vi "1.0.2_UUT_Reflashing.vi"(8 "error in (no error)":errorcluster, 10 "Data in":T1, 11 "Message Queue out":T2) -> (0 "error out":errorcluster, 1 "Flow":string, 2 "Data out":T1, 3 "Message Queue Out":T2)   [LabVIEW 2017]
uses:
  Depends/AMC/subVIs/TypeDefs/amc_Message Queue.ctl
  Depends/AMC/subVIs/TypeDefs/amc_Message.ctl
  Depends/Tools/Keyed Array/Tools_KeyedArray KeyedArray.ctl
  Ctrls/CSV_Data.ctl
  DIPC 692 Daemon API/typdef/destination.ctl
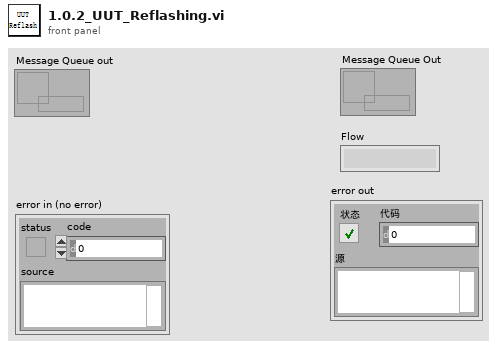
[diagram p1: front panel]
types:
  T1 = typedef "CSV_Data.ctl" = cluster{"Initialisation":cluster{"LMT - Connect UUT (con COM)":string, "LMT - Software Version (rrel)":string, "LMT - Write SKU file (wskuc)":string, "LMT - SKU file name":string, "Connect UUT DDM":string, "Read DDM EOL Timestamp - Mode":string, "Read DDM EOL Timestamp - Timestamp":string, "Read DDM EOL Timestamp - Rig ID":string, "Read DDM EOL Timestamp - Passmark ID":string, "Read DDM EOL Timestamp - Passmark Rev":string, "Software Version before flashing":string, "Read Hardware Serial":string, "UUT DDM SN":string, "Compare DDM SN with MES SN":string, "Backup PCBA Calibration EEPROM Response - CAL":string, "Flash Firmware Version":string, "Check SW Version":string, "Read DDM SW Version after flashing":string, "Set SKU Config":string, "Ready Status":string, "Set Device Mode to EOL":string, "DDM Parameter - Voltage":string, "DDM Parameter - Current":string, "DDM Parameter - Power":string, "DDM Parameter - Speed":string, "DDM Parameter - Pressure":string, "Tester Parameter - Voltage":string, "Tester Parameter - Current":string, "Tester Parameter - Power":string, "Tester Parameter - Ambient Pressure":string, "Tester Parameter - Ambient Temperature":string, "Calculated Parameter - DDM Pressure Corrected":string, "Calculated Parameter - DDM Real Power":string, "Calculated Parameter - Delta V":string}, "BEMF_Calibration":cluster{"Calibration Result - eol_cold_bemf_temp":string, "DDM Ambient Temp":string, "Restriction Plate Diameter":string, "Calibration Result - eol_bemf_mp_cold_coef_a":string, "Calibration Result - eol_bemf_mp_cold_coef_b":string, "Calibration Result - eol_bemf_mp_cold_coef_c":string, "Calibration Result - eol_bemf_lsi_cold_ref_coeffs":string, "Get - Calibration Result - eol_bemf_lsi_speed":string, "Get - Calibration Result - eol_bemf_lsi_integral_0":string, "Calibration Result - eol_bemf_lsi_integral_1":string, "Get - Calibration Result - eol_bemf_lsi_integral_2":string, "Get - Calibration Result - eol_cold_bemf":string, "Get - Calibration Result - eol_cold_bemf_fisf":string, "Finalise Calibration":string, "Compare -Calibration Result - eol_cold_bemf":string, "Compare -Calibration Result - eol_cold_bemf_fisf":string}, "ECO":cluster{"Reset Power Tune":string, "Reset BEMF FISF Calibration":string, "Restriction Plate Diameter":string, "ECO - Stabilisation Time":string, "ECO - DDM Parameter - Voltage":string, "ECO - DDM Parameter - Current":string, "ECO - DDM Parameter - Power":string, "ECO - DDM Parameter - Measured Power":string, "ECO - DDM Parameter - Speed":string, "ECO - DDM Parameter - Pressure":string, "ECO - Tester Parameter - Voltage":string, "ECO - Tester Parameter - Current":string, "ECO - Tester Parameter - Power":string, "ECO - Tester Parameter - Ambient Pressure":string, "ECO - Tester Parameter - Ambient Temperature":string, "ECO - Tester Parameter - Ambient Humidity":string, "ECO - Calculated Parameter - DDM Pressure Corrected":string, "ECO - Calculated Parameter - DDM Real Power":string, "ECO - Calculated Parameter - Delta V":string, "ECO - Calculated Parameter - Flowrate":string, "ECO - Calculated Parameter - Airwatt":string, "ECO - Formula":string, "PT ECO - Power Tune Mode Status":string}, "BOOST":cluster{"Restriction Plate Diameter":string, "BOOST - Stabilisation Time":string, "BOOST - DDM Parameter - Voltage":string, "BOOST - DDM Parameter - Current":string, "BOOST - DDM Parameter - Power":string, "BOOST - DDM Parameter - Measured Power":string, "BOOST - DDM Parameter - Speed":string, "BOOST - DDM Parameter - Pressure":string, "BOOST - Tester Parameter - Voltage":string, "BOOST - Tester Parameter - Current":string, "BOOST - Tester Parameter - Power":string, "BOOST - Tester Parameter - Ambient Pressure":string, "BOOST - Tester Parameter - Ambient Temperature":string, "BOOST - Tester Parameter - Ambient Humidity":string, "BOOST - Calculated Parameter - DDM Pressure Corrected":string, "BOOST - Calculated Parameter - DDM Real Power":string, "BOOST - Calculated Parameter - Delta V":string, "BOOST - Calculated Parameter - Flowrate":string, "BOOST - Calculated Parameter - Airwatt":string, "BOOST - Get AM Presence":string, "Air Muscle Turn Off Status":string, "BOOST - Air Muscle Calculated Parameter - Airwatt B":string, "BOOST - Air Muscle Calculate Airwatt Delta":string, "PT BOOST - Power Tune Mode Status":string, "Finalise Calibration":string, "ECO - Get AW Calibration value":string, "BOOST - Get AW Calibration value":string}, "MAX":cluster{"Restriction Plate Diameter":string, "MAX - Stabilisation Time":string, "Get Average Delta Tmag (LSIdelta_FISFdelta_LSItmag_FISFtmag_IIRtmag)":string, "Get Average Delta Tmag FISF":string, "MAX - DDM Parameter - Voltage":string, "MAX - DDM Parameter - Current":string, "MAX - DDM Parameter - Power":string, "MAX - DDM Parameter - Measured Power":string, "MAX - DDM Parameter - Speed":string, "MAX - DDM Parameter - Pressure":string, "MAX - Tester Parameter - Voltage":string, "MAX - Tester Parameter - Current":string, "MAX - Tester Parameter - Power":string, "MAX - Tester Parameter - Ambient Pressure":string, "MAX - Tester Parameter - Ambient Temperature":string, "MAX - Tester Parameter - Ambient Humidity":string, "MAX - Calculated Parameter - DDM Pressure Corrected":string, "MAX - Calculated Parameter - DDM Real Power":string, "MAX - Calculated Parameter - Delta V":string, "MAX - Calculated Parameter - Flowrate":string, "MAX - Calculated Parameter - Airwatt":string, "MAX_FISF_Check_Average_Delta_Tmag":string, "MAX - FISF - BEMF Finetune Result":string, "MAX tune - Delta P1":string, "MAX tune - Calculated Parameter - Airwatt":string, "Calculate Delta Airwatts - MAX finetune - Delta P2":string, "MAX finetune - DDM Parameter - Voltage":string, "MAX finetune - DDM Parameter - Current":string, "MAX finetune - DDM Parameter - Power":string, "MAX finetune - DDM Parameter - Measured Power":string, "MAX finetune - DDM Parameter - Speed":string, "MAX finetune - DDM Parameter - Pressure":string, "MAX finetune - Tester Parameter - Voltage":string, "MAX finetune - Tester Parameter - Current":string, "MAX finetune - Tester Parameter - Power":string, "MAX finetune - Tester Parameter - Ambient Pressure":string, "MAX finetune - Tester Parameter - Ambient Temperature":string, "MAX finetune - Tester Parameter - Ambient Humidity":string, "MAX finetune - Calculated Parameter - DDM Pressure Corrected":string, "MAX finetune - Calculated Parameter - DDM Real Power":string, "MAX finetune - Calculated Parameter - Delta V":string, "MAX finetune - Calculated Parameter - Flowrate":string, "MAX finetune - Calculated Parameter - Airwatt":string, "Check Derate Result":string, "Delta Tmag FISF":string, "Get Hot BEMF Result":string, "Calculate delta Pressure":string, "Finalise Calibration":string, "Calculate & Check Delta BEMF":string, "Delta P Airwatts Value":string}, "LL":cluster{"DDM Ambient Temp":string, "Restriction Plate Diameter":string, "LL - DDM Parameter - Voltage":string, "LL - DDM Parameter - Current":string, "LL - DDM Parameter - Power":string, "LL - DDM Parameter - Measured Power":string, "LL - DDM Parameter - Speed":string, "LL - DDM Parameter - Pressure":string, "LL - Tester Parameter - Voltage":string, "LL - Tester Parameter - Current":string, "LL - Tester Parameter - Power":string, "LL - DDM Real Power":string, "LL - Calibrate Task Detect LL":string}, "HL":cluster{"HL - DDM Parameter - Voltage":string, "HL - DDM Parameter - Current":string, "HL - DDM Parameter - Power":string, "HL - DDM Parameter - Measured Power":string, "HL - DDM Parameter - Speed":string, "HL - DDM Parameter - Pressure":string, "HL - Tester Parameter - Voltage":string, "HL - Tester Parameter - Current":string, "HL - Tester Parameter - Power":string, "HL - DDM Real Power":string, "HL - Calibrate Task Detect HL":string}, "LH":cluster{"Restriction Plate Diameter":string, "LH - DDM Parameter - Voltage":string, "LH - DDM Parameter - Current":string, "LH - DDM Parameter - Power":string, "LH - DDM Parameter - Measured Power":string, "LH - DDM Parameter - Speed":string, "LH - DDM Parameter - Pressure":string, "LH - Tester Parameter - Voltage":string, "LH - Tester Parameter - Current":string, "LH - Tester Parameter - Power":string, "LH - DDM Real Power":string, "LH - Calibrate Task Detect LH":string}, "HH":cluster{"HH - DDM Parameter - Voltage":string, "HH - DDM Parameter - Current":string, "HH - DDM Parameter - Power":string, "HH - DDM Parameter - Measured Power":string, "HH - DDM Parameter - Speed":string, "HH - DDM Parameter - Pressure":string, "HH - Tester Parameter - Voltage":string, "HH - Tester Parameter - Current":string, "HH - Tester Parameter - Power":string, "HH - DDM Real Power":string, "HH - Calibrate Task Detect HH":string}, "Inlet Blockage Calibration":cluster{"Inlet Blockage Calibration - DDM Parameter - Voltage":string, "Inlet Blockage Calibration - DDM Parameter - Current":string, "Inlet Blockage Calibration - DDM Parameter - Power":string, "Inlet Blockage Calibration - DDM Parameter - Measured Power":string, "Inlet Blockage Calibration - DDM Parameter - Speed":string, "Inlet Blockage Calibration - DDM Parameter - Pressure":string, "Inlet Blockage Calibration - Tester Parameter - Voltage":string, "Inlet Blockage Calibration - Tester Parameter - Current":string, "Inlet Blockage Calibration - Tester Parameter - Power":string, "Inlet Blockage Calibration - DDM Real Power":string, "Calibration Inlet Blockage_E":string, "Finalise Calibration":string, "Get Task Detect LL":string, "Get Task Detect HL":string, "Get Task Detect LH":string, "Get Task Detect HH":string, "Calibration Inlet Blockage":string, "Calibration eol cold bemf temp":string}, "GOOD":cluster{"GOOD UNIT - Clear EEPROM Error Log":string, "GOOD UNIT - Write Product Timestamp - Mode":string, "GOOD UNIT - Write Product Timestamp - Timestamp":string, "GOOD UNIT - Write Product Timestamp - Rig ID":string, "GOOD UNIT - Write Product Timestamp - Passmark ID":string, "GOOD UNIT - Write Product Timestamp - Passmark Rev":string, "GOOD UNIT - Set Device Mode to PROD":string, "GOOD UNIT - Backup PCBA Calibration EEPROM Response":string, "GOOD UNIT - Check Security Bit":string, "GOOD UNIT - Set Calibration Lock":string, "GOOD UNIT - Get_Calibration_Lock":string, "GOOD UNIT - Disconnect UUT":string}, "NG":cluster{"NG UNIT - Read NVM Error":string, "NG UNIT - Set Device Mode to FCT":string, "NG UNIT - Backup PCBA Calibration EEPROM Response - CAL":string, "NG UNIT - Backup PCBA Calibration EEPROM Response - ERROR":string, "NG UNIT - Backup PCBA Calibration EEPROM Response - USAGE":string, "NG UNIT - Disconnect UUT":string}, "SN":string, "Table":string[][], "Count":cluster{"Total":i32, "OK":i32, "NG":i32, "Yield":dbl}, "Start Time":timestamp, "daemon reference":refnum<k5>, "CT":dbl, "Config":string[][], "OK/NG":bool, "Station ID":string, "MES DDM SN":string, "MES PCBA SN":string, "Retest":string, "Lux":string, "Initialisation_Status":cluster{"LMT - Connect UUT (con COM)":string, "LMT - Software Version (rrel)":string, "LMT - Write SKU file (wskuc)":string, "LMT - SKU file name":string, "Connect UUT DDM":string, "Read DDM EOL Timestamp - Mode":string, "Read DDM EOL Timestamp - Timestamp":string, "Read DDM EOL Timestamp - Rig ID":string, "Read DDM EOL Timestamp - Passmark ID":string, "Read DDM EOL Timestamp - Passmark Rev":string, "Software Version before flashing":string, "Read Hardware Serial":string, "UUT DDM SN":string, "Compare DDM SN with MES SN":string, "Backup PCBA Calibration EEPROM Response - CAL":string, "Flash Firmware Version":string, "Check SW Version":string, "Read DDM SW Version after flashing":string, "Set SKU Config":string, "Ready Status":string, "Set Device Mode to EOL":string, "DDM Parameter - Voltage":string, "DDM Parameter - Current":string, "DDM Parameter - Power":string, "DDM Parameter - Speed":string, "DDM Parameter - Pressure":string, "Tester Parameter - Voltage":string, "Tester Parameter - Current":string, "Tester Parameter - Power":string, "Tester Parameter - Ambient Pressure":string, "Tester Parameter - Ambient Temperature":string, "Calculated Parameter - DDM Pressure Corrected":string, "Calculated Parameter - DDM Real Power":string, "Calculated Parameter - Delta V":string}, "BEMF_Calibration_Status":cluster{"Calibration Result - eol_cold_bemf_temp":string, "DDM Ambient Temp":string, "Restriction Plate Diameter":string, "Calibration Result - eol_bemf_mp_cold_coef_a":string, "Calibration Result - eol_bemf_mp_cold_coef_b":string, "Calibration Result - eol_bemf_mp_cold_coef_c":string, "Calibration Result - eol_bemf_lsi_cold_ref_coeffs":string, "Get - Calibration Result - eol_bemf_lsi_speed":string, "Get - Calibration Result - eol_bemf_lsi_integral_0":string, "Calibration Result - eol_bemf_lsi_integral_1":string, "Get - Calibration Result - eol_bemf_lsi_integral_2":string, "Get - Calibration Result - eol_cold_bemf":string, "Get - Calibration Result - eol_cold_bemf_fisf":string, "Finalise Calibration":string, "Compare -Calibration Result - eol_cold_bemf":string, "Compare -Calibration Result - eol_cold_bemf_fisf":string}, "ECO_Status":cluster{"Reset Power Tune":string, "Reset BEMF FISF Calibration":string, "Restriction Plate Diameter":string, "ECO - Stabilisation Time":string, "ECO - DDM Parameter - Voltage":string, "ECO - DDM Parameter - Current":string, "ECO - DDM Parameter - Power":string, "ECO - DDM Parameter - Measured Power":string, "ECO - DDM Parameter - Speed":string, "ECO - DDM Parameter - Pressure":string, "ECO - Tester Parameter - Voltage":string, "ECO - Tester Parameter - Current":string, "ECO - Tester Parameter - Power":string, "ECO - Tester Parameter - Ambient Pressure":string, "ECO - Tester Parameter - Ambient Temperature":string, "ECO - Tester Parameter - Ambient Humidity":string, "ECO - Calculated Parameter - DDM Pressure Corrected":string, "ECO - Calculated Parameter - DDM Real Power":string, "ECO - Calculated Parameter - Delta V":string, "ECO - Calculated Parameter - Flowrate":string, "ECO - Calculated Parameter - Airwatt":string, "ECO - Formula":string, "PT ECO - Power Tune Mode Status":string}, "BOOST_Status":cluster{"Restriction Plate Diameter":string, "BOOST - Stabilisation Time":string, "BOOST - DDM Parameter - Voltage":string, "BOOST - DDM Parameter - Current":string, "BOOST - DDM Parameter - Power":string, "BOOST - DDM Parameter - Measured Power":string, "BOOST - DDM Parameter - Speed":string, "BOOST - DDM Parameter - Pressure":string, "BOOST - Tester Parameter - Voltage":string, "BOOST - Tester Parameter - Current":string, "BOOST - Tester Parameter - Power":string, "BOOST - Tester Parameter - Ambient Pressure":string, "BOOST - Tester Parameter - Ambient Temperature":string, "BOOST - Tester Parameter - Ambient Humidity":string, "BOOST - Calculated Parameter - DDM Pressure Corrected":string, "BOOST - Calculated Parameter - DDM Real Power":string, "BOOST - Calculated Parameter - Delta V":string, "BOOST - Calculated Parameter - Flowrate":string, "BOOST - Calculated Parameter - Airwatt":string, "BOOST - Get AM Presence":string, "Air Muscle Turn Off Status":string, "BOOST - Air Muscle Calculated Parameter - Airwatt B":string, "BOOST - Air Muscle Calculate Airwatt Delta":string, "PT BOOST - Power Tune Mode Status":string, "Finalise Calibration":string, "ECO - Get AW Calibration value":string, "BOOST - Get AW Calibration value":string}, "MAX_Status":cluster{"Restriction Plate Diameter":string, "MAX - Stabilisation Time":string, "Get Average Delta Tmag (LSIdelta_FISFdelta_LSItmag_FISFtmag_IIRtmag)":string, "Get Average Delta Tmag FISF":string, "MAX - DDM Parameter - Voltage":string, "MAX - DDM Parameter - Current":string, "MAX - DDM Parameter - Power":string, "MAX - DDM Parameter - Measured Power":string, "MAX - DDM Parameter - Speed":string, "MAX - DDM Parameter - Pressure":string, "MAX - Tester Parameter - Voltage":string, "MAX - Tester Parameter - Current":string, "MAX - Tester Parameter - Power":string, "MAX - Tester Parameter - Ambient Pressure":string, "MAX - Tester Parameter - Ambient Temperature":string, "MAX - Tester Parameter - Ambient Humidity":string, "MAX - Calculated Parameter - DDM Pressure Corrected":string, "MAX - Calculated Parameter - DDM Real Power":string, "MAX - Calculated Parameter - Delta V":string, "MAX - Calculated Parameter - Flowrate":string, "MAX - Calculated Parameter - Airwatt":string, "MAX_FISF_Check_Average_Delta_Tmag":string, "MAX - FISF - BEMF Finetune Result":string, "MAX tune - Delta P1":string, "MAX tune - Calculated Parameter - Airwatt":string, "Calculate Delta Airwatts - MAX finetune - Delta P2":string, "MAX finetune - DDM Parameter - Voltage":string, "MAX finetune - DDM Parameter - Current":string, "MAX finetune - DDM Parameter - Power":string, "MAX finetune - DDM Parameter - Measured Power":string, "MAX finetune - DDM Parameter - Speed":string, "MAX finetune - DDM Parameter - Pressure":string, "MAX finetune - Tester Parameter - Voltage":string, "MAX finetune - Tester Parameter - Current":string, "MAX finetune - Tester Parameter - Power":string, "MAX finetune - Tester Parameter - Ambient Pressure":string, "MAX finetune - Tester Parameter - Ambient Temperature":string, "MAX finetune - Tester Parameter - Ambient Humidity":string, "MAX finetune - Calculated Parameter - DDM Pressure Corrected":string, "MAX finetune - Calculated Parameter - DDM Real Power":string, "MAX finetune - Calculated Parameter - Delta V":string, "MAX finetune - Calculated Parameter - Flowrate":string, "MAX finetune - Calculated Parameter - Airwatt":string, "Check Derate Result":string, "Delta Tmag FISF":string, "Get Hot BEMF Result":string, "Calculate delta Pressure":string, "Finalise Calibration":string, "Calculate & Check Delta BEMF":string, "Delta P Airwatts Value":string}, "LL_Status":cluster{"DDM Ambient Temp":string, "Restriction Plate Diameter":string, "LL - DDM Parameter - Voltage":string, "LL - DDM Parameter - Current":string, "LL - DDM Parameter - Power":string, "LL - DDM Parameter - Measured Power":string, "LL - DDM Parameter - Speed":string, "LL - DDM Parameter - Pressure":string, "LL - Tester Parameter - Voltage":string, "LL - Tester Parameter - Current":string, "LL - Tester Parameter - Power":string, "LL - DDM Real Power":string, "LL - Calibrate Task Detect LL":string}, "HL_Status":cluster{"HL - DDM Parameter - Voltage":string, "HL - DDM Parameter - Current":string, "HL - DDM Parameter - Power":string, "HL - DDM Parameter - Measured Power":string, "HL - DDM Parameter - Speed":string, "HL - DDM Parameter - Pressure":string, "HL - Tester Parameter - Voltage":string, "HL - Tester Parameter - Current":string, "HL - Tester Parameter - Power":string, "HL - DDM Real Power":string, "HL - Calibrate Task Detect HL":string}, "LH_Status":cluster{"Restriction Plate Diameter":string, "LH - DDM Parameter - Voltage":string, "LH - DDM Parameter - Current":string, "LH - DDM Parameter - Power":string, "LH - DDM Parameter - Measured Power":string, "LH - DDM Parameter - Speed":string, "LH - DDM Parameter - Pressure":string, "LH - Tester Parameter - Voltage":string, "LH - Tester Parameter - Current":string, "LH - Tester Parameter - Power":string, "LH - DDM Real Power":string, "LH - Calibrate Task Detect LH":string}, "HH_Status":cluster{"HH - DDM Parameter - Voltage":string, "HH - DDM Parameter - Current":string, "HH - DDM Parameter - Power":string, "HH - DDM Parameter - Measured Power":string, "HH - DDM Parameter - Speed":string, "HH - DDM Parameter - Pressure":string, "HH - Tester Parameter - Voltage":string, "HH - Tester Parameter - Current":string, "HH - Tester Parameter - Power":string, "HH - DDM Real Power":string, "HH - Calibrate Task Detect HH":string}, "Inlet Blockage Calibration_Status":cluster{"Inlet Blockage Calibration - DDM Parameter - Voltage":string, "Inlet Blockage Calibration - DDM Parameter - Current":string, "Inlet Blockage Calibration - DDM Parameter - Power":string, "Inlet Blockage Calibration - DDM Parameter - Measured Power":string, "Inlet Blockage Calibration - DDM Parameter - Speed":string, "Inlet Blockage Calibration - DDM Parameter - Pressure":string, "Inlet Blockage Calibration - Tester Parameter - Voltage":string, "Inlet Blockage Calibration - Tester Parameter - Current":string, "Inlet Blockage Calibration - Tester Parameter - Power":string, "Inlet Blockage Calibration - DDM Real Power":string, "Calibration Inlet Blockage_E":string, "Finalise Calibration":string, "Get Task Detect LL":string, "Get Task Detect HL":string, "Get Task Detect LH":string, "Get Task Detect HH":string, "Calibration Inlet Blockage":string, "Calibration eol cold bemf temp":string}, "GOOD_Status":cluster{"GOOD UNIT - Clear EEPROM Error Log":string, "GOOD UNIT - Write Product Timestamp - Mode":string, "GOOD UNIT - Write Product Timestamp - Timestamp":string, "GOOD UNIT - Write Product Timestamp - Rig ID":string, "GOOD UNIT - Write Product Timestamp - Passmark ID":string, "GOOD UNIT - Write Product Timestamp - Passmark Rev":string, "GOOD UNIT - Set Device Mode to PROD":string, "GOOD UNIT - Backup PCBA Calibration EEPROM Response":string, "GOOD UNIT - Check Security Bit":string, "GOOD UNIT - Set Calibration Lock":string, "GOOD UNIT - Get_Calibration_Lock":string, "GOOD UNIT - Disconnect UUT":string}, "NG_Status":cluster{"NG UNIT - Read NVM Error":string, "NG UNIT - Set Device Mode to FCT":string, "NG UNIT - Backup PCBA Calibration EEPROM Response - CAL":string, "NG UNIT - Backup PCBA Calibration EEPROM Response - ERROR":string, "NG UNIT - Backup PCBA Calibration EEPROM Response - USAGE":string, "NG UNIT - Disconnect UUT":string}, "SKU":string, "Plate_Diameter":string, "Alarm":string}
  T2 = typedef "amc_Message Queue.ctl" = refnum<queue>
  T3 = typedef "HD Config.ctl" = cluster{" PC":cluster{"PC Address":u8[], "PC Port":i32}, "FCO":cluster{"COM":refnum<visa-resource-name>, "Baudrate":u32}, "DC Power ":cluster{"COM":refnum<visa-resource-name>, "Baudrate":u32}, "PW3336":cluster{"COM":refnum<visa-resource-name>, "Baudrate":u32}, "Lefoo":cluster{"COM":refnum<visa-resource-name>, "Baudrate":u32}, "Tempt&Hum":cluster{"COM":refnum<visa-resource-name>, "Baudrate":u32}, "DIPC":cluster{"COM":refnum<visa-resource-name>}, "Daemon":cluster{"IP Address":string, "Port":u16, "Retry":u16}, "NFC":cluster{"COM":refnum<visa-resource-name>, "Baudrate":u32}, "Fail_resume_mode":bool, "GRR":bool}
  T4 = typedef "destination.ctl" = string
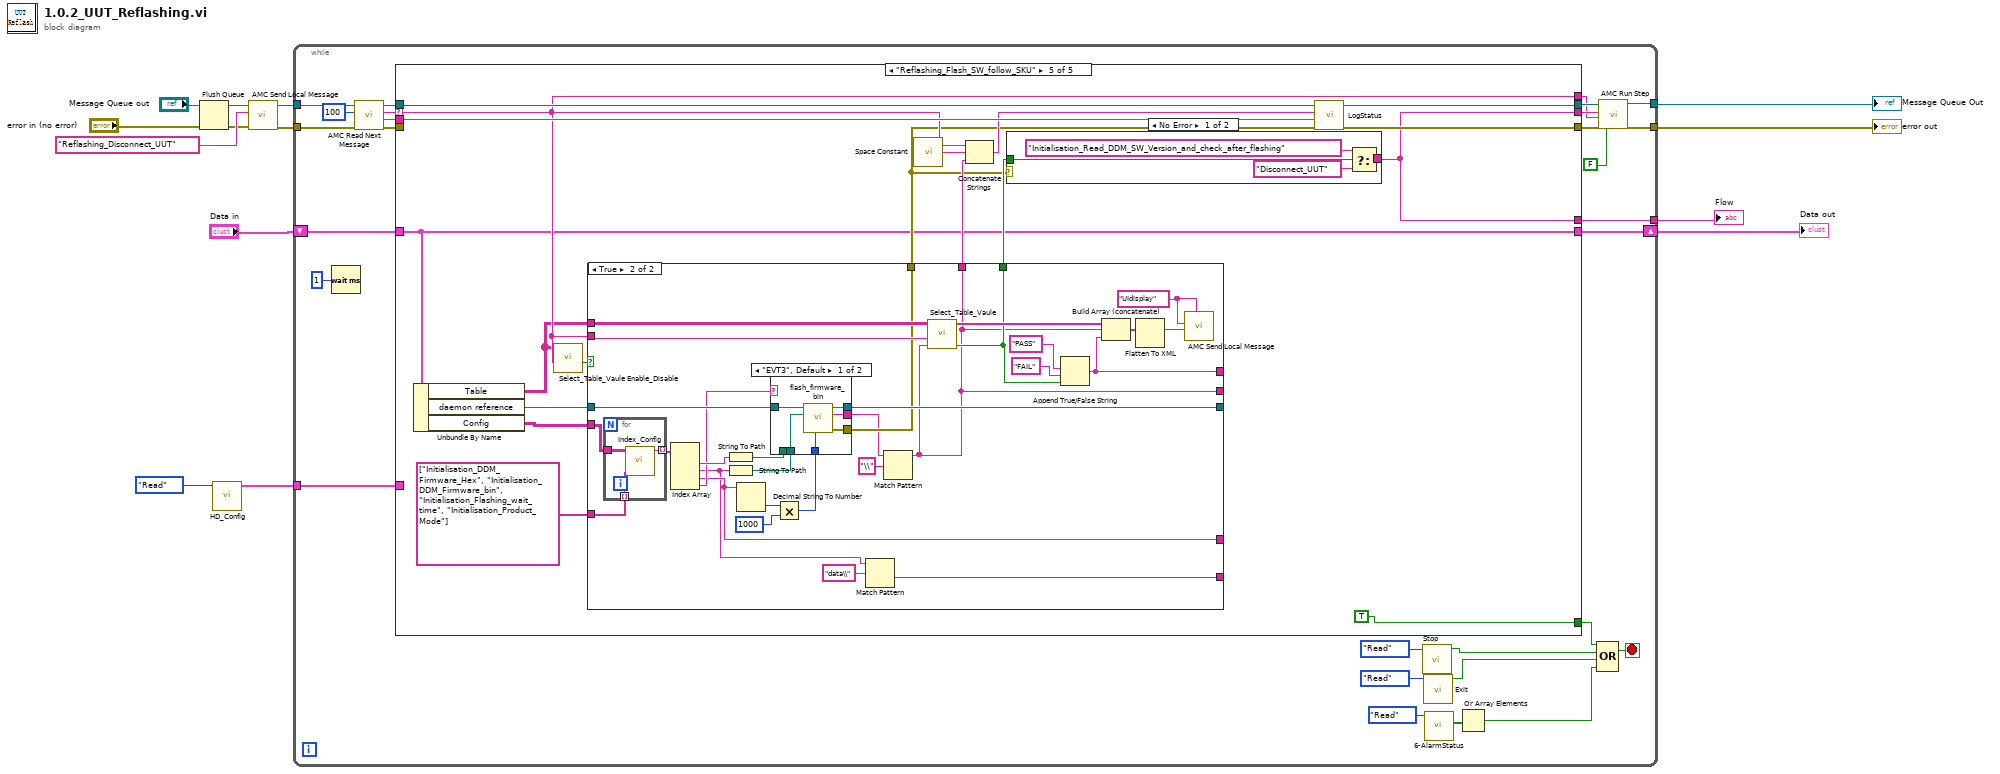
[diagram p0: block diagram]
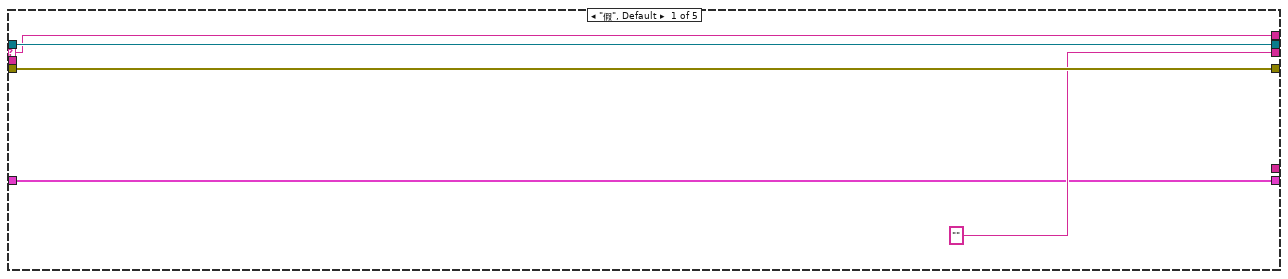
[diagram p2: hidden frame]
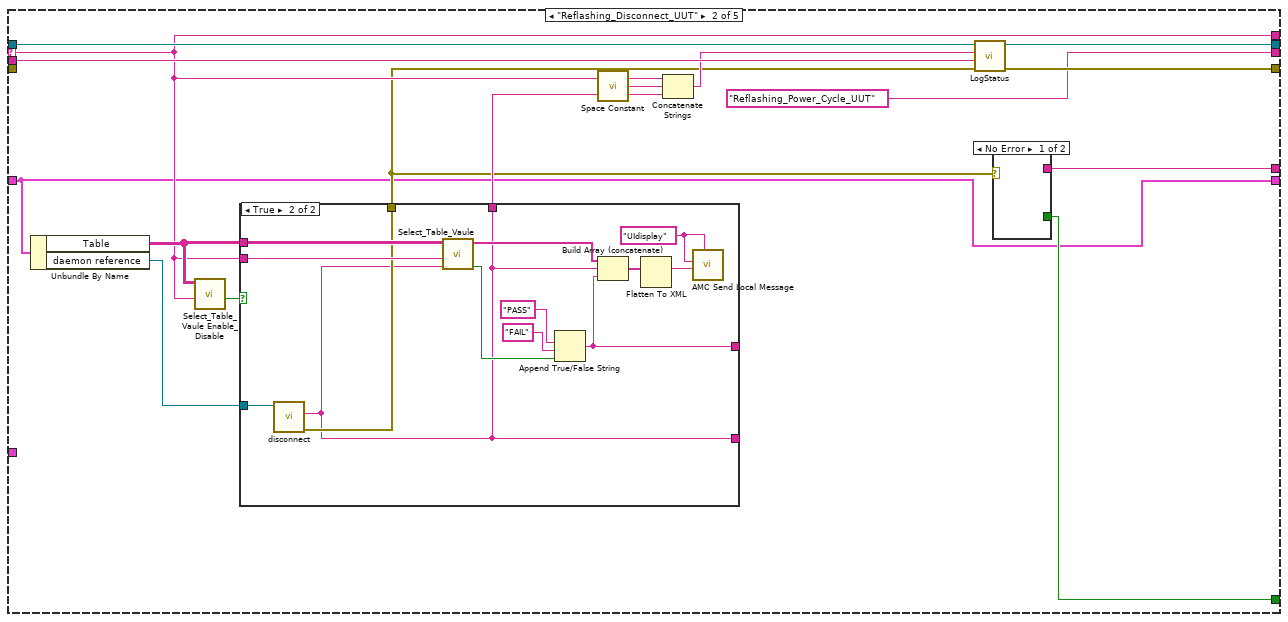
[diagram p3: hidden frame]
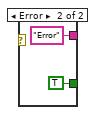
[diagram p4: hidden frame]
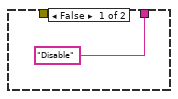
[diagram p5: hidden frame]
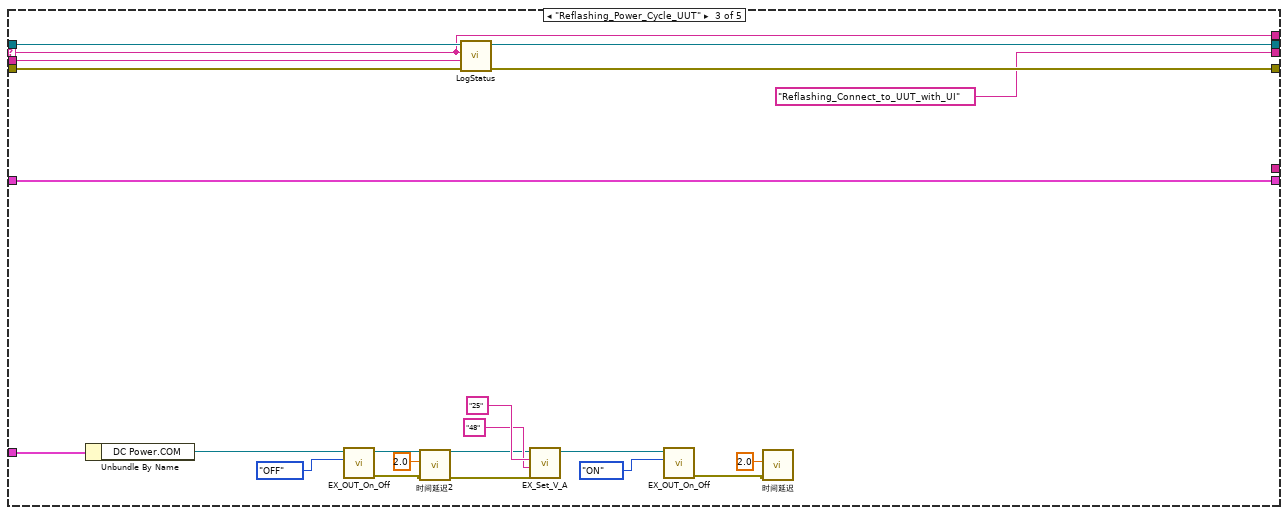
[diagram p6: hidden frame]
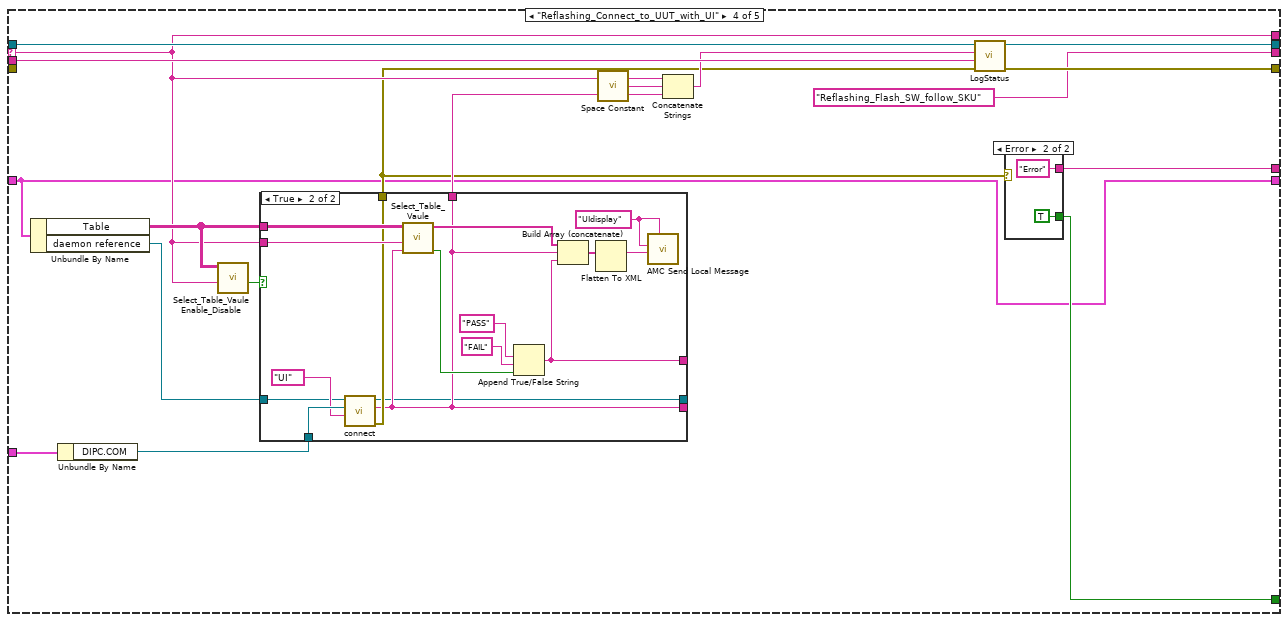
[diagram p7: hidden frame]
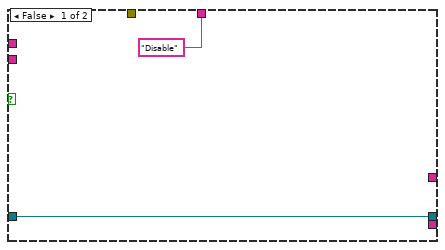
[diagram p9: hidden frame]
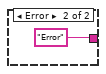
[diagram p10: hidden frame]
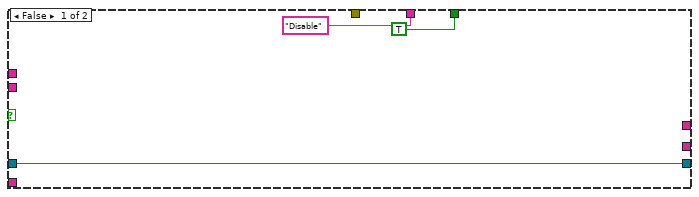
[diagram p11: hidden frame]
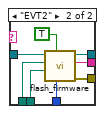
[diagram p12: hidden frame]
diagram:
  n1 = Flush Queue(queue="Message Queue out") -> (queue out=w5:T2)  [unwired: 1 in, 2 out]
  n2 = call "HD_Config.vi"("Step"=enum16{"Initial", "Write", "Read"}."Read") -> ("HD Config out"=w7:T3)  [unwired: 9 in, 1 out]
  n3 = call "AMC Send Local Message.vi"("error in (no error)"="error in (no error)", "Message Name"="Reflashing_Disconnect_UUT", "Message Queue in"=w5) -> ("error out"=w10:errorcluster, "Message Queue out"=w11:T2)  [unwired: 7 in]
  n4 = while {
    tunnel: w11 -> [w41]
    tunnel: [w37] -> w4
    tunnel: w10 -> [w35]
    tunnel: [w32] -> w3
    tunnel: w7 -> [w29]
    tunnel: [w25] -> w6
    shift-right: [w17] -> w1
    shift-left: "Data in" -> [w18]
    stop <- w19 stop-if-true
    n5 = Wait (ms)(milliseconds to wait=u32 1 ("等待时间（毫秒）")) -> ()  [unwired: 1 out]
    n6 = call "AMC Read Next Message.vi"("error in (no error)"=w35, "timeout (1ms)"=100, "Message Queue in"=w41) -> ("error out"=w34:errorcluster, "Message Value"=w27:string, "Message Name"=w39:string, "Message Queue out"=w40:T2)  [unwired: 1 in, 4 out]
    n7 = case shown="\"Reflashing_Flash_SW_follow_SKU\"" w39 {
      selector: w39 -> [w44 w53 w93 w104 w145]
      tunnel: w40 -> [w46 w61 w97 w114 w151]
      tunnel: [w46 w61 w97 w114 w151] -> w38
      tunnel: w34 -> [w45 _ w96 _ _]
      tunnel: [w45 w60 w95 w113 w150] -> w33
      tunnel: [_ w49 _ w101 TRUE] -> w20
      tunnel: w27 -> [_ w59 w94 w112 w149]
      tunnel: [w44 w53 w93 w104 w145] -> w26
      tunnel: w29 -> [_ _ w87 w110 _]
      tunnel: ["" "Reflashing_Power_Cycle_UUT" "Reflashing_Connect_to_UUT_with_UI" "Reflashing_Flash_SW_follow_SKU" w139] -> w28
      tunnel: [_ w50 _ w102 w139] -> w25
      tunnel: w18 -> [w42 w47 w81 w98 w135]
      tunnel: [w42 w47 w81 w98 w135] -> w17
      frame "假", Default {
      }
      frame "Reflashing_Disconnect_UUT" {
        n8 = Unbundle By Name(w47) -> ("Table"=w54:string[][], "daemon reference"=w51:refnum<k5>)
        n9 = call "Select_Table_Vaule Enable_Disable.vi"("Action"=w53, "Table"=w54) -> ("Enable"=w52:bool)  [unwired: 8 in, 1 out]
        n10 = case shown="True" w52 {
          tunnel: ["Disable" ("response") w66] -> w55
          tunnel: w54 -> [_ w70]
          tunnel: w53 -> [_ w69]
          tunnel: w51 -> [_ w68]
          tunnel: [_ w67] -> w48
          tunnel: [_ w66] -> _
          tunnel: [_ w65] -> _
          frame False {
          }
          frame True {
            w76 = "UIdisplay" ("Process (\"\" - local)")
            n11 = call "disconnect.vi"("daemon reference in"=w68) -> ("error out"=w67:errorcluster, "response"=w66:string)  [unwired: 7 in, 2 out]
            n12 = call "Select_Table_Vaule.vi"("Vaule"=w66, "Action"=w69, "Table"=w70) -> ("Result"=w71:bool, "vaule"=w77:string[])  [unwired: 7 in]
            n13 = Append True/False String(1:w71, 2:"FAIL" ("真字符串"), 3:"PASS" ("真字符串")) -> (0:w65:string)  [unwired: 1 in]
            n14 = Build Array (concatenate)(w77, w66, w65) -> (w75:string[])
            n15 = Flatten To XML(anything=w75) -> (xml string=w74:string)
            n16 = call "AMC Send Local Message.vi"("Process (\"\" - local)"=w76, "Message Value"=w74, "Message Name"=w76) -> ()  [unwired: 7 in, 2 out]
          }
        }
        n17 = call <vilib>:"Space Constant.vi"() -> ("String"=w56:string)
        n18 = Concatenate Strings(w53, w56, w55) -> (w57:string)
        n19 = call "LogStatus.vi"("error in (no error)"=w48, "last message"=w59, "message"=w57) -> ("error  out"=w60:errorcluster)  [unwired: 8 in]
        n20 = case shown="No Error" w48 {
          tunnel: [_ TRUE] -> w49
          tunnel: [_ "Error"] -> w50
          frame No Error {
          }
          frame Error {
          }
        }
      }
      frame "Reflashing_Power_Cycle_UUT" {
        n21 = Unbundle By Name(w87) -> ("DC Power.COM"=w85:refnum<visa-resource-name>)
        n22 = call "EX_OUT_On_Off.vi"("Mode"=enum16{"ON", "OFF"}."OFF", "VISA resource name"=w85) -> ("error out"=w79:errorcluster, "VISA资源名称输出"=w84:refnum<visa-resource-name>)  [unwired: 8 in]
        n23 = call "时间延迟2"("error in (no error)"=w79, "Delay Time (s)"=2.0) -> ("error out"=w78:errorcluster)  [unwired: 9 in]
        n24 = call "LogStatus.vi"("error in (no error)"=w96, "last message"=w94, "message"=w93) -> ("error  out"=w95:errorcluster)  [unwired: 8 in]
        n25 = call "EX_Set_V_A.vi"("错误输入（无错误）"=w78, "current"="48", "voltage"="25", "VISA resource name"=w84) -> ("VISA资源名称输出"=w89:refnum<visa-resource-name>)  [unwired: 6 in, 1 out]
        n26 = call "EX_OUT_On_Off.vi"("Mode"=enum16{"ON", "OFF"}."ON", "VISA resource name"=w89) -> ("error out"=w83:errorcluster)  [unwired: 8 in, 1 out]
        n27 = call "时间延迟"("error in (no error)"=w83, "Delay Time (s)"=2.0) -> ()  [unwired: 9 in, 1 out]
      }
      frame "Reflashing_Connect_to_UUT_with_UI" {
        n28 = Unbundle By Name(w98) -> ("Table"=w105:string[][], "daemon reference"=w100:refnum<k5>)
        n29 = Unbundle By Name(w110) -> ("DIPC.COM"=w109:refnum<visa-resource-name>)
        n30 = call "Select_Table_Vaule Enable_Disable.vi"("Action"=w104, "Table"=w105) -> ("Enable"=w103:bool)  [unwired: 8 in, 1 out]
        n31 = case shown="True" w103 {
          tunnel: w109 -> [_ w134]
          tunnel: ["Disable" ("response") w121] -> w106
          tunnel: w105 -> [_ w126]
          tunnel: w104 -> [_ w125]
          tunnel: [_ w123] -> w99
          tunnel: w100 -> [w117 w122]
          tunnel: [_ w121] -> _
          tunnel: [w117 w120] -> _
          tunnel: [_ w119] -> _
          frame False {
          }
          frame True {
            w132 = "UIdisplay" ("Process (\"\" - local)")
            n32 = call "connect.vi"("Target"=T4 "UI", "physical connection"=w134, "daemon reference in"=w122) -> ("error out"=w123:errorcluster, "response"=w121:string, "daemon reference out"=w120:refnum<k5>)  [unwired: 4 in, 2 out]
            n33 = call "Select_Table_Vaule.vi"("Vaule"=w121, "Action"=w125, "Table"=w126) -> ("Result"=w127:bool, "vaule"=w133:string[])  [unwired: 7 in]
            n34 = Append True/False String(1:w127, 2:"FAIL" ("真字符串"), 3:"PASS" ("真字符串")) -> (0:w119:string)  [unwired: 1 in]
            n35 = Build Array (concatenate)(w133, w121, w119) -> (w131:string[])
            n36 = Flatten To XML(anything=w131) -> (xml string=w130:string)
            n37 = call "AMC Send Local Message.vi"("Process (\"\" - local)"=w132, "Message Value"=w130, "Message Name"=w132) -> ()  [unwired: 7 in, 2 out]
          }
        }
        n38 = call <vilib>:"Space Constant.vi"() -> ("String"=w107:string)
        n39 = Concatenate Strings(w104, w107, w106) -> (w108:string)
        n40 = call "LogStatus.vi"("error in (no error)"=w99, "last message"=w112, "message"=w108) -> ("error  out"=w113:errorcluster)  [unwired: 8 in]
        n41 = case shown="Error" w99 {
          tunnel: [_ TRUE] -> w101
          tunnel: [_ "Error"] -> w102
          frame No Error {
          }
          frame Error {
          }
        }
      }
      frame "Reflashing_Flash_SW_follow_SKU" {
        n42 = Unbundle By Name(w135) -> ("Table"=w144:string[][], "daemon reference"=w148:refnum<k5>, "Config"=w142:string[][])
        n43 = call "Select_Table_Vaule Enable_Disable.vi"("Action"=w145, "Table"=w144) -> ("Enable"=w143:bool)  [unwired: 8 in, 1 out]
        n44 = case shown="True" w143 {
          tunnel: w148 -> [w159 w184]
          tunnel: [w159 w183] -> _
          tunnel: ["Disable" ("software string") w165] -> w138
          tunnel: w145 -> [_ w182]
          tunnel: w144 -> [_ w181]
          tunnel: w142 -> [_ w171]
          tunnel: [TRUE w179] -> w140
          tunnel: string[] ["Initialisation_DDM_Firmware_Hex", "Initialisation_DDM_Firmware_bin", "Initialisation_Flashing_wait_time", "Initialisation_Product_Mode"] -> [_ w170]
          tunnel: [_ w169] -> w136
          tunnel: [_ w165] -> _
          tunnel: [_ w164] -> _
          tunnel: [_ w163] -> _
          tunnel: [_ w160] -> _
          frame False {
          }
          frame True {
            w189 = "UIdisplay" ("Process (\"\" - local)")
            n45 = for {
              tunnel: w171 -> [w206]
              tunnel: w170 -> [w205] mode=indexing
              tunnel: [w204] -> w176 mode=indexing
              n46 = call "Index_Config.vi"("Action"=w205, "config"=w206) -> ("data"=w204:string)  [unwired: 9 in]
            }
            n47 = Index Array(array=w176) -> (element #1=w177:string, element #2=w161:string, element #3=w163:string, element #4=w166:string)  [unwired: 4 in]
            n48 = String To Path(string=w177) -> (path=w174:path)
            n49 = String To Path(string=w161) -> (path=w173:path)
            n50 = Decimal String To Number(string=w163) -> (number=w178:i32)  [unwired: 2 in, 1 out]
            n51 = Multiply(x=w178, y=1000) -> (x*y=w172:i32)
            n52 = case shown="\"EVT3\", Default" w166 {
              tunnel: w184 -> [w194 w203]
              tunnel: [w195 w202] -> w183
              tunnel: w174 -> [_ w200]
              tunnel: w173 -> [w193 w199]
              tunnel: w172 -> [w192 w198]
              tunnel: [w191 w197] -> w169
              tunnel: [w190 w196] -> w167
              frame "EVT3", Default {
                n53 = call "flash_firmware_bin.vi"("timeout (25000ms)"=w192, "firmware path"=w193, "daemon reference in"=w194) -> ("error out"=w191:errorcluster, "response"=w190:string, "daemon reference out"=w195:refnum<k5>)  [unwired: 5 in, 1 out]
              }
              frame "EVT2" {
                n54 = call "flash_firmware.vi"("timeout (25000ms)"=w198, "SW 4.1 and above?"=TRUE, "SIV bin path"=w199, "firmware path"=w200, "daemon reference in"=w203) -> ("error out"=w197:errorcluster, "response"=w196:string, "daemon reference out"=w202:refnum<k5>)  [unwired: 3 in, 1 out]
              }
            }
            n55 = Match Pattern(string=w161, regular expression="data\\") -> (after substring=w160:string)  [unwired: 1 in, 3 out]
            n56 = Match Pattern(string=w167, regular expression="\\") -> (before substring=w165:string)  [unwired: 1 in, 3 out]
            n57 = call "Select_Table_Vaule.vi"("Vaule"=w165, "Action"=w182, "Table"=w181) -> ("Result"=w179:bool, "vaule"=w180:string[])  [unwired: 7 in]
            n58 = Append True/False String(1:w179, 2:"FAIL" ("真字符串"), 3:"PASS" ("真字符串")) -> (0:w164:string)  [unwired: 1 in]
            n59 = Build Array (concatenate)(w180, w165, w164) -> (w188:string[])
            n60 = Flatten To XML(anything=w188) -> (xml string=w187:string)
            n61 = call "AMC Send Local Message.vi"("Process (\"\" - local)"=w189, "Message Value"=w187, "Message Name"=w189) -> ()  [unwired: 7 in, 2 out]
          }
        }
        n62 = call <vilib>:"Space Constant.vi"() -> ("String"=w147:string)
        n63 = Concatenate Strings(w145, w147, w138) -> (w146:string)
        n64 = case shown="No Error" w136 {
          tunnel: w140 -> [w155 _]
          tunnel: [w152 "Error"] -> w139
          frame No Error {
            n65 = Select(t="Initialisation_Read_DDM_SW_Version_and_check_after_flashing", s=w155, f="Disconnect_UUT") -> (s? t:f=w152:string)
          }
          frame Error {
          }
        }
        n66 = call "LogStatus.vi"("error in (no error)"=w136, "last message"=w149, "message"=w146) -> ("error  out"=w150:errorcluster)  [unwired: 8 in]
      }
    }
    n67 = call "Stop.vi"("Step"=enum16{"Initial", "Write", "Read"}."Read") -> ("Stop Out"=w22:bool)  [unwired: 9 in, 1 out]
    n68 = call "Exit.vi"("Step"=enum16{"Initial", "Write", "Read"}."Read" ("step")) -> ("Exit Out"=w21:bool)  [unwired: 9 in, 1 out]
    n69 = call "6-AlarmStatus.vi"("Step"=enum16{"Initial", "Write", "Read"}."Read") -> ("AlarmValue Out"=w15:bool[])  [unwired: 9 in, 1 out]
    n70 = Or Array Elements(Boolean array=w15) -> (logical OR=w14:bool)
    n71 = Compound Arithmetic op=OR(w20, w22, w21, w14) -> (w19:bool)
    n72 = call "AMC Run Step.vi"("Message Queue In"=w38, "Message Name"=w28, "Message Value"=w26, "error in (no error)"=w33, "Mli/Sig"=FALSE) -> ("Message Queue Out"=w37:T2, "error out"=w32:errorcluster)  [unwired: 13 in]
  }
  "Message Queue Out" <- w4
  "error out" <- w3
  "Flow" <- w6
  "Data out" <- w1
